vi "Error.vi"(8 "error in (no error)":errorcluster, 10 "error":errorcluster, 11 "~Error in":refnum<class "~Error.lvclass">) -> (0 "error out":errorcluster, 3 "~Error out":refnum<class "~Error.lvclass">)   [LabVIEW 2024, in "Error Reporting Actor.lvlib" / "~Error.lvlib" / "~Error.lvclass"]
uses:
  ~Error.lvclass
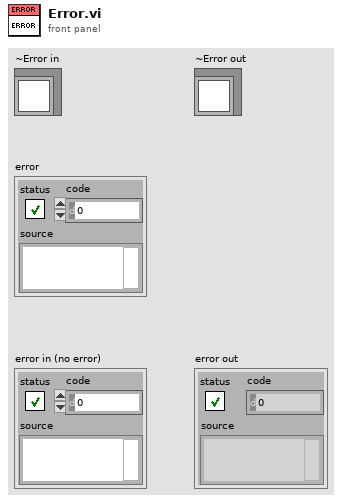
[diagram p1: front panel]
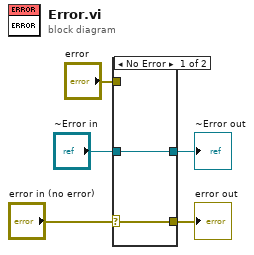
[diagram p0: block diagram]
diagram:
  n1 = case shown="No Error" "error in (no error)" {
    selector: "error in (no error)" -> [w6 w9]
    tunnel: [w6 w9] -> w4
    tunnel: [w7 w8] -> w2
    tunnel: "~Error in" -> [w7 w8]
    tunnel: "error" -> [_ _]
    frame No Error {
    }
    frame Error {
    }
  }
  "error out" <- w4
  "~Error out" <- w2
